vi "SetDataTrFreq.vi"(8 "错误输入（无错误）":errorcluster, 11 "数据传输率":sgl) -> (0 "错误输出":errorcluster)   [LabVIEW 2018]
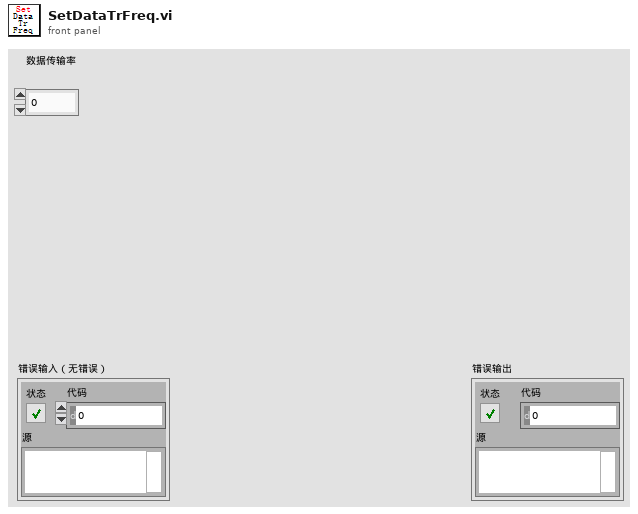
[diagram p1: front panel]
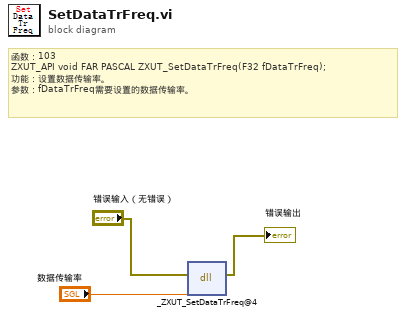
[diagram p0: block diagram]
diagram:
  # "函数：103\nZXUT_API void\tFAR PASCAL ZXUT_SetDataTrFreq(F32 fDataTrFreq);\n功能：设置数据传输率。\n参数：fDataTrFreq需要设置的数据传输率。"
  n1 = dll-call lib="PTH2Rabs E软件项目超声超声子VI函数VI\tTCG处理ZXUTConfigMgr.dll" fn="_ZXUT_SetDataTrFreq@4"(error in="错误输入（无错误）", "fDataTrFreq"="数据传输率") -> (error out=→"错误输出":errorcluster)  [unwired: 4 in, 1 out]
